vi "InterpolateCircle.vi"(2 "Radius":dbl, 3 "Start Angle (degrees)":dbl, 4 "Number of Points":u32) -> (0 "Y coordinates":dbl[](array[numeric]), 1 "X coordinates":dbl[](array[numeric]))   [LabVIEW 2011]
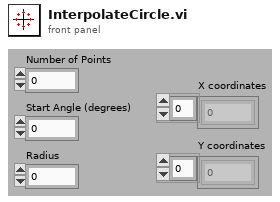
[diagram p1: front panel]
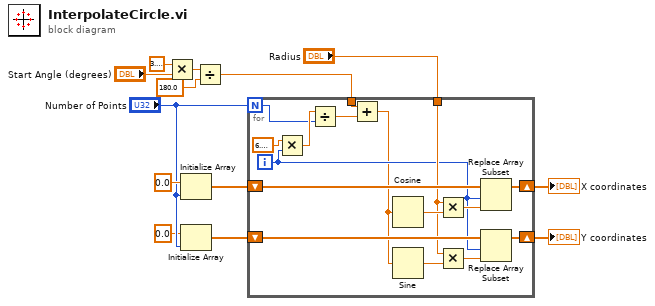
[diagram p0: block diagram]
diagram:
  n1 = Multiply(x=3.141592653589793, y="Start Angle (degrees)") -> (x*y=w5:dbl)
  n2 = Initialize Array(0.0 ("element"), "Number of Points") -> (w10:dbl[])
  n3 = Initialize Array(0.0 ("element"), "Number of Points") -> (w9:dbl[])
  n4 = Divide(x=w5, y=180.0) -> (x/y=w1:dbl)
  n5 = for {
    N: "Number of Points" -> [w16]
    shift-right: [w28] -> w8
    shift-left: w10 -> [w29]
    shift-right: [w26] -> w7
    shift-left: w9 -> [w21]
    tunnel: "Radius" -> [w20]
    tunnel: w1 -> [w14]
    i -> [w19]
    n6 = Multiply(x=6.283185307179586, y=w19) -> (x*y=w17:dbl)
    n7 = Divide(x=w17, y=w16) -> (x/y=w15:dbl)
    n8 = Add(x=w14, y=w15) -> (x+y=w18:dbl)
    n9 = Cosine(x=w18) -> (cos(x)=w24:dbl)
    n10 = Sine(x=w18) -> (sin(x)=w23:dbl)
    n11 = Multiply(x=w20, y=w24) -> (x*y=w25:dbl)
    n12 = Multiply(x=w20, y=w23) -> (x*y=w22:dbl)
    n13 = Replace Array Subset(array=w29, new element=w25, index=w19) -> (w28:dbl[])
    n14 = Replace Array Subset(array=w21, new element=w22, index=w19) -> (w26:dbl[])
  }
  "X coordinates" <- w8
  "Y coordinates" <- w7
